vi "数据查询_调试数据.vi"() -> ()   [LabVIEW 2016]
uses:
  <vilib>/Utility/miscctls.llb/LVRowAndColumnUnsignedTypeDef.ctl
  <vilib>/Utility/sysdir.llb/System Directory Type.ctl
  <vilib>/Utility/miscctls.llb/LVPointTypeDef.ctl
  <vilib>/addons/database/Connection.llb/DB Tools Open Connec (String).vi
  <vilib>/addons/database/NI_Database_API.lvlib
panel:
  out "选中数据表":string
  in  "查询":bool
  in  "结束日期":string="2020/01/01"
  in  "起始日期":string="2010/01/01"
  in  "组合框":string(combo)
  out "数据表":string[][](table)
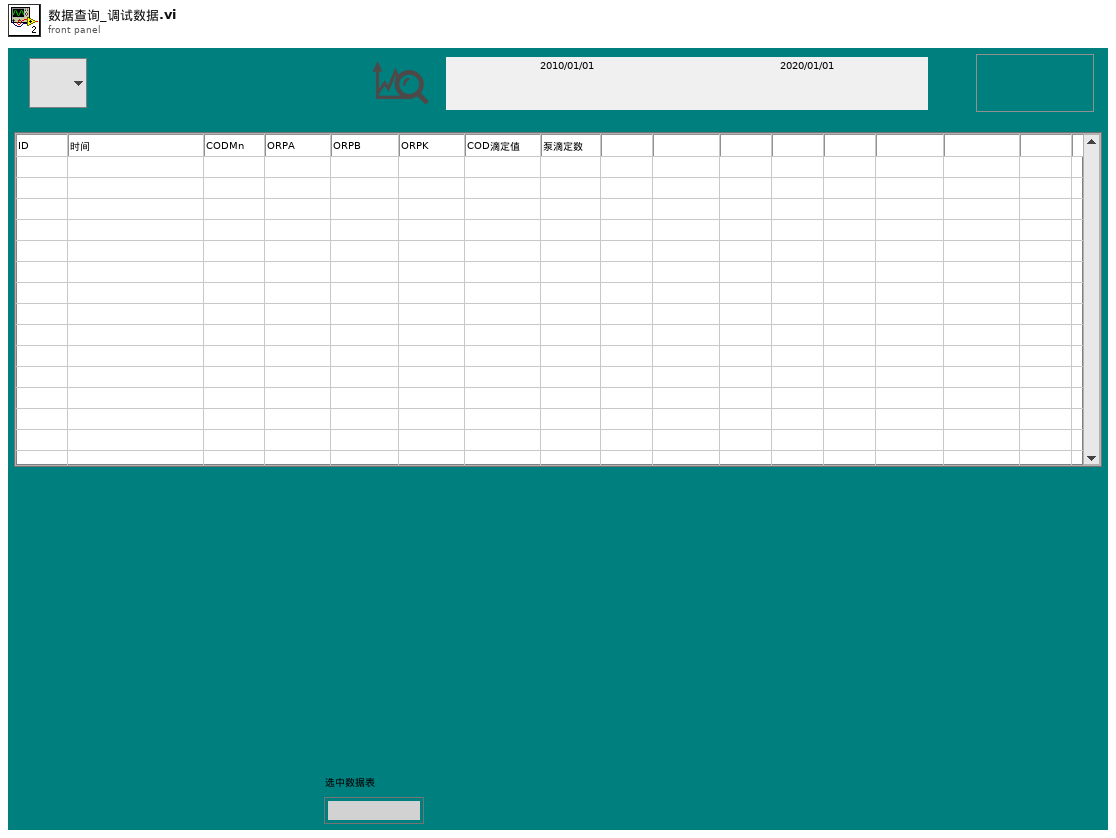
[diagram p1: front panel]
types:
  T1 = typedef "LVRowAndColumnUnsignedTypeDef.ctl" = cluster{"Row":u32, "Column":u32}
  T2 = typedef "LVPointTypeDef.ctl" = cluster{"Horizontal":i16, "Vertical":i16}
  T3 = typedef "System Directory Type.ctl" = i32
  T4 = typedef "NI_Database_API.lvlib/Conn ObjectReference.ctl" = refnum<k1>
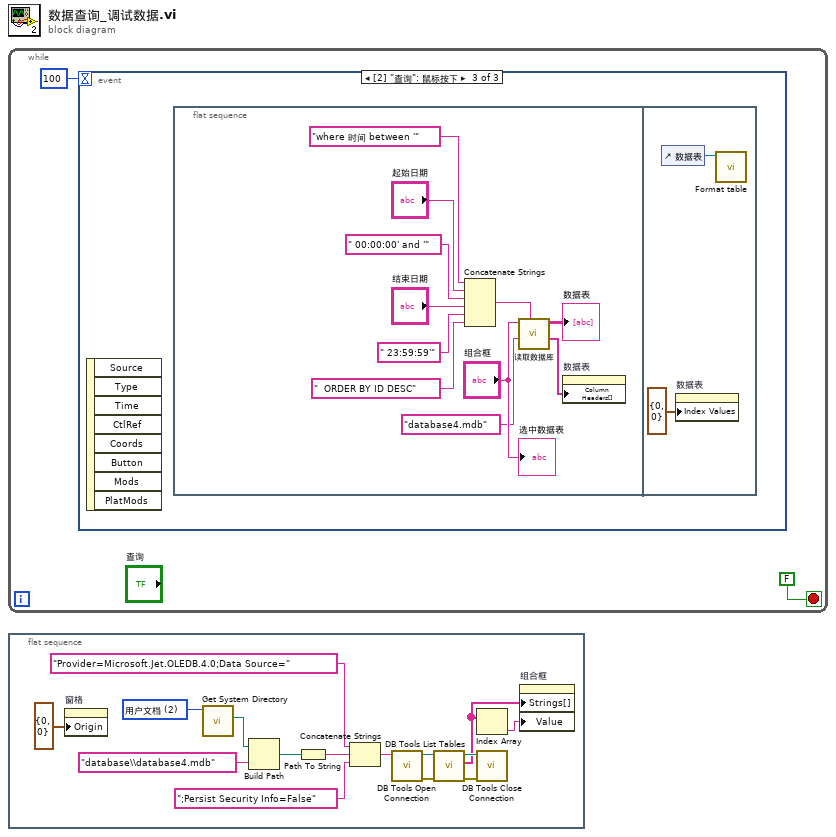
[diagram p0: block diagram]
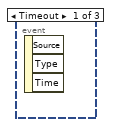
[diagram p2: hidden frame]
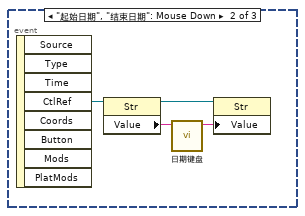
[diagram p3: hidden frame]
diagram:
  n1 = while {
    stop <- FALSE stop-if-true
    n2 = event shown="[2] \"查询\": 鼠标按下" {
      selector: _ -> [_ _ _]
      dyn-events: _ -> [_ _ _]
      timeout: 100 -> [_ _ _]
      event Timeout {
        n3 = event-data() -> ()  [unwired: 1 in, 3 out]
      }
      event "起始日期", "结束日期": Mouse Down {
        n4 = event-data() -> ("CtlRef"=w6:refnum<vi>)  [unwired: 1 in, 7 out]
        n5 = property class="Str"(reference=w6) -> (reference out=w4:refnum<vi>, "Value"=w5:string)  [unwired: 1 in, 1 out]
        n6 = call "日期键盘.vi"("原值"=w5) -> ("x+y"=w3:string)  [unwired: 10 in]
        n7 = property class="Str"(reference=w4, "Value"=w3) -> ()  [unwired: 1 in, 2 out]
      }
      event "查询": Mouse Down {
        n8 = event-data() -> ()  [unwired: 1 in, 8 out]
        n9 = flat-sequence {
          frame #0 {
            n10 = Concatenate Strings("where 时间 between '" ("condition"), "起始日期", " 00:00:00' and '" ("condition"), "结束日期", " 23:59:59'" ("condition"), "  ORDER BY ID DESC" ("字符串")) -> (w16:string)
            n11 = call "读取数据库.vi"("condition"=w16, "database"="database4.mdb", "组合框"="组合框") -> ("columns"=w10:string[], "表格"=→"数据表":string[][])  [unwired: 5 in, 2 out]
            n12 = property on="数据表" class="Tbl (严格)"("Column Headers[]"=w10) -> ()  [unwired: 2 in, 2 out]
            "选中数据表" <- "组合框"
          }
          frame #1 {
            n13 = control-ref of="数据表"() -> (w19:refnum<vi>)
            n14 = property on="数据表" class="Tbl (严格)"("Index Values"=T1 {"Row"=0, "Column"=0} ("索引值")) -> ()  [unwired: 2 in, 2 out]
            n15 = call "Format table.vi"("Table输入"=w19) -> ()  [unwired: 11 in]
          }
        }
      }
    }
  }
  n16 = flat-sequence {
    frame #0 {
      w30 = T3 2 items=["用户目录"=0, "用户桌面"=1, "用户文档"=2, "用户应用程序数据"=3, "用户设置"=4, "用户临时目录"=5, "公共文档"=6, "公共应用程序数据"=7, "公共设置"=8, "公共缓存"=13, "系统核心库"=9, "系统安装库"=10, "应用程序文件"=11, "启动盘根目录"=12] ("system directory type")
      n17 = property on="窗格" class="Pane"("Origin"=T2 {"Horizontal"=0, "Vertical"=0} ("原点")) -> ()  [unwired: 2 in, 2 out]
      n18 = call <vilib>:"Get System Directory.vi"("system directory type"=w30) -> ("system directory"=w29:path)  [unwired: 10 in]
      n19 = Build Path(base path=w29, name or relative path="database\\database4.mdb" ("名称或相对路径")) -> (appended path=w31:path)
      n20 = Path To String(path=w31) -> (string=w32:string)
      n21 = Concatenate Strings("Provider=Microsoft.Jet.OLEDB.4.0;Data Source=", w32, ";Persist Security Info=False") -> (w28:string)
      n22 = call-poly <vilib>:"DB Tools Open Connection.vi"("connection information"=w28) -> ("error out"=w25:errorcluster, "connection reference"=w26:T4)  [unwired: 7 in]
      n23 = call <vilib>:"DB Tools List Tables.vi"("error in (no error)"=w25, "connection reference"=w26) -> ("error out"=w23:errorcluster, "tables"=w22:string[], "connection reference out"=w24:T4)  [unwired: 3 in]
      n24 = Index Array(array=w22) -> (element=w21:string)  [unwired: 1 in]
      n25 = call <vilib>:"DB Tools Close Connection.vi"("error in (no error)"=w23, "connection reference"=w24) -> ()  [unwired: 5 in, 1 out]
      n26 = property on="组合框" class="CmbBox"("Strings[]"=w22, "Value"=w21) -> ()  [unwired: 2 in, 2 out]
    }
  }
